vi "XML_StripContent.vi"(8 "Tag":string="ObjXMLNode", 11 "XML":T1="<ObjXMLNode>\n  <ModuleName>WaveformGen</ModuleName>\n  <ObjName>WaveformGen</ObjName>\n<Terminal Name=\"WaveformGen.Waveform\" TerminalType=\"Output\">\n<ObjXMLNode>\n  <ModuleName>WaveformDisplay</ModuleName>\n  <ObjName>Display1</ObjName>\n</ObjXMLNode>\n<ObjXMLNode>\n  <ModuleName>WaveformStreaming</ModuleName>\n  <ObjName>Streaming</ObjName>\n</ObjXMLNode>\n<ObjXMLNode>\n  <ModuleName>WaveformFFT</ModuleName>\n  <ObjName>WaveformFFT</ObjName>\n<Terminal Name=\"WaveformFFT.FFT\" TerminalType=\"Output\">\n<ObjXMLNode>\n  <ModuleName>WaveformDisplay</ModuleName>\n  <ObjName>Display3</ObjName>\n</ObjXMLNode>\n</Terminal>\n</ObjXMLNode>\n<ObjXMLNode>\n  <ModuleName>WaveformHistoryCache</ModuleName>\n  <ObjName>WaveformHistoryCache</ObjName>\n<Terminal Name=\"WaveformHistoryCache.HistoryCache\" TerminalType=\"Output\">\n<ObjXMLNode>\n  <ModuleName>WaveformDisplay</ModuleName>\n  <ObjName>Display2</ObjName>\n</ObjXMLNode>\n</Terminal>\n</ObjXMLNode>\n</Terminal>\n</ObjXMLNode>") -> (2 "Left":T1, 3 "Content":T1)   [LabVIEW 2017]
doc: "Removes the element named Tag from XML and returns the content of that element separately."
uses:
  _XML--String.ctl
panel:
  out "offset (0)":i32
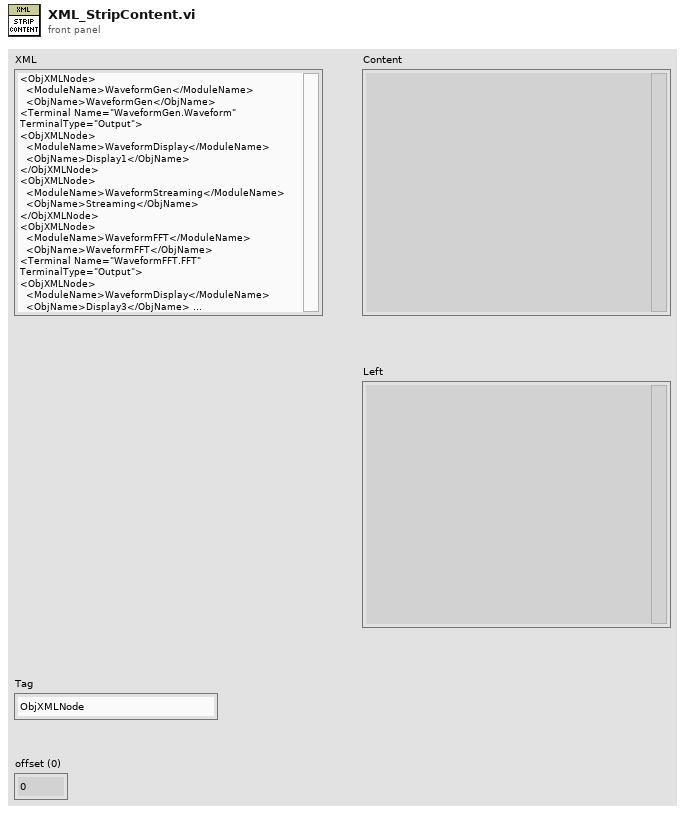
[diagram p1: front panel]
types:
  T1 = typedef "_XML--String.ctl" = string
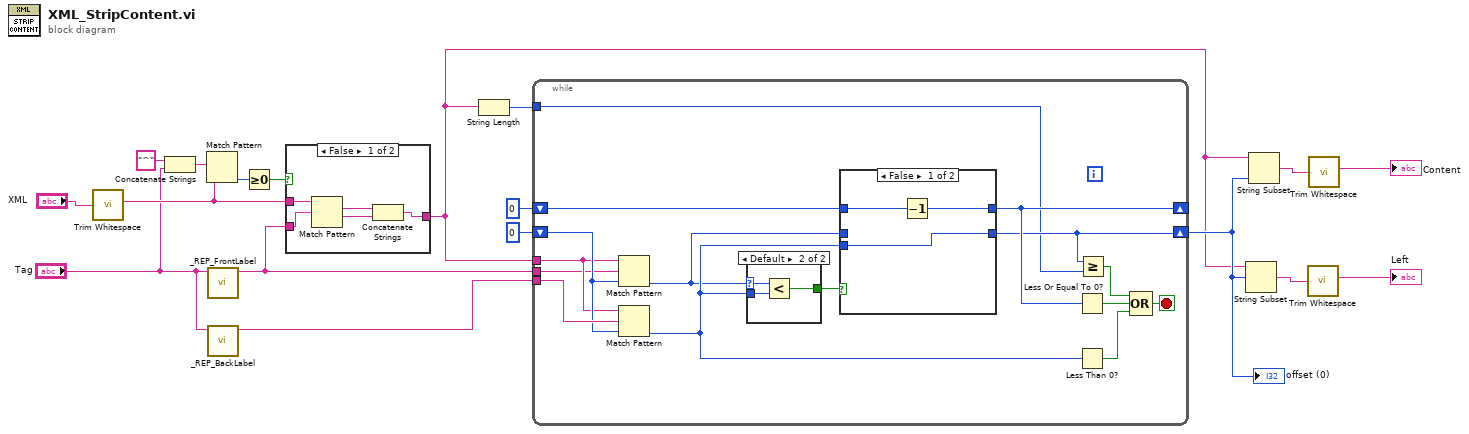
[diagram p0: block diagram]
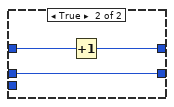
[diagram p4: hidden frame]
diagram:
  n1 = call <vilib>:"Trim Whitespace.vi"("string"="XML") -> ("trimmed string"=w6:string)  [unwired: 1 in]
  n2 = Concatenate Strings("^" ("string"), "Tag") -> (w5:string)
  n3 = Match Pattern(string=w6, regular expression=w5) -> (offset past match=w2:i32)  [unwired: 1 in, 3 out]
  n4 = call "_REP_FrontLabel.vi"("label"="Tag") -> ("String"=w8:string)  [unwired: 10 in]
  n5 = call "_REP_BackLabel.vi"("label"="Tag") -> ("String"=w16:string)  [unwired: 10 in]
  n6 = Greater Or Equal To 0?(x=w2) -> (x >= 0?=w1:bool)
  n7 = case shown="False" w1 {
    tunnel: w8 -> [w23 _]
    tunnel: [w20 w24] -> w7
    tunnel: w6 -> [w21 w24]
    frame False {
      n8 = Match Pattern(string=w21, regular expression=w23) -> (match substring=w19:string, after substring=w22:string)  [unwired: 1 in, 2 out]
      n9 = Concatenate Strings(w19, w22) -> (w20:string)
    }
    frame True {
    }
  }
  n10 = String Length(string=w7) -> (length=w13:i32)
  n11 = while {
    tunnel: w7 -> [w30]
    shift-right: [w33] -> w12
    shift-left: 0 ("offset (0)") -> [w38]
    tunnel: w8 -> [w27]
    tunnel: w16 -> [w39]
    shift-right: [w36] -> _
    shift-left: 0 ("offset (0)") -> [w37]
    tunnel: w13 -> [w31]
    stop <- w34 stop-if-true
    n12 = Match Pattern(string=w30, regular expression=w27, offset (0)=w38) -> (offset past match=w25:i32)  [unwired: 3 out]
    n13 = Match Pattern(string=w30, regular expression=w39, offset (0)=w38) -> (offset past match=w29:i32)  [unwired: 3 out]
    n14 = case shown="Default" w25 {
      selector: w25 -> [_ w41]
      tunnel: w29 -> [_ w42]
      tunnel: [_ w40] -> w26
      frame ..-1 {
      }
      frame Default {
        n15 = Less?(x=w41, y=w42) -> (x < y?=w40:bool)
      }
    }
    n16 = case shown="False" w26 {
      tunnel: [w44 w47] -> w36
      tunnel: w37 -> [w45 w48]
      tunnel: w25 -> [_ w46]
      tunnel: w29 -> [w43 _]
      tunnel: [w43 w46] -> w33
      frame False {
        n17 = Decrement(x=w45) -> (x-1=w44:i32)
      }
      frame True {
        n18 = Increment(x=w48) -> (x+1=w47:i32)
      }
    }
    n19 = Less Or Equal To 0?(x=w36) -> (x <= 0?=w35:bool)
    n20 = Less Than 0?(x=w29) -> (x < 0?=w28:bool)
    n21 = Greater Or Equal?(x=w33, y=w31) -> (x >= y?=w32:bool)
    n22 = Compound Arithmetic op=OR(w32, w35, w28) -> (w34:bool)
  }
  "offset (0)" <- w12
  n23 = String Subset(string=w7, offset (0)=w12) -> (substring=w11:string)  [unwired: 1 in]
  n24 = String Subset(string=w7, length (rest)=w12) -> (substring=w10:string)  [unwired: 1 in]
  n25 = call <vilib>:"Trim Whitespace.vi"("string"=w11) -> ("trimmed string"=→"Left":string)  [unwired: 1 in]
  n26 = call <vilib>:"Trim Whitespace.vi"("string"=w10) -> ("trimmed string"=→"Content":string)  [unwired: 1 in]
